vi "Online Spectrogram Monitoring (DAQmx).vi"() -> ()   [LabVIEW 2023]
doc: "This example shows how to configure a DAQ device, continuously acquire data from the specified physical channel with given sampling rate, and compute the real-time STFT spectrogram with the TFA Online STFT Spectrogram VI.\n\n<b>Requirements:</b>\nThis example requires a DAQ device and NI-DAQmx driver.\n\n<b>Instructions:</b>\n1) Select the data acquisition channel and sampling rate.\n2) Set the parameters for the STFT.\n3) Run this VI.\n4) Observe what frequencies are in your signal from the spectrogram.\n5) Browse the Block Diagram to learn how to configure the charts and how to connect TFA VIs with DAQmx VIs."
uses:
  <vilib>/DAQmx/read.llb/DAQmx Read (Analog 1D DBL 1Chan NSamp).vi
  <vilib>/DAQmx/create/channels.llb/DAQmx Create Channel (AI-Acceleration-Accelerometer).vi
  <vilib>/DAQmx/configure/timing.llb/DAQmx Timing (Sample Clock).vi
  <vilib>/DAQmx/miscellaneous.llb/DAQmx Fill In Error Info.vi
  <vilib>/addons/Time Frequency Analysis/Spectrogram.llb/TFA Online STFT Spectrogram (Real).vi
  <vilib>/addons/Time Frequency Analysis/_control.llb/TFA Configure Spectrogram Indicator (Predefined Color Table).vi
  <vilib>/addons/_Advanced Signal Processing/NI_AdvSigProcTFA.lvlib
  <resource>/objmgr/daqmx.rc
panel:
  out "aspt-left-top":bool
  in  "Window info":cluster{"type":u16, "length":i32}={"type"=0, "length"=256} {"type" items=["None ", "Hanning", "Hamming", "Blackman-Harris", "Exact Blackman", "Blackman", "Flat Top", "4 Term B-Harris ", "7 Term B-Harris", "Low Sidelobe", "Gaussian"]}
  in  "dB?":bool
  in  "Stop":bool
  in  "Sampling rate (Hz)":dbl=10000.0 format="%.2f"
  in  "Channel":tag="Dev2/ai0"
  in  "Frequency bins":i32=512
  in  "Time steps":i32=64
  out "Signal":dbl[](graph)
  out "Spectrogram":dbl[][](graph)
  # "Overview: Shows how to configure a DAQ device,  continuously acquire data from the specified physical channel with given sampling rate, and compute the real-time STFT spectrogram with the TFA Online STFT Spectrogram VI.\nRequirements: LabVIEW Full Development System, Advanced Signal Processing Toolkit, DAQmx Device\nInstructions: \n1. Select the data acquisition channel and sampling rate.\n2. Set the parameters for the STFT.\n3. Run this VI.\n4. Observe what frequencies are in your signal from the spectrogram.\n5. Browse the block diagram to learn how to configure the charts and how to connect TFA VIs with DAQmx VIs.\n6. Click Stop to stop the VI."
  # "Hardware Settings"
  # "Signal and Spectrogram"
  # "STFT Settings"
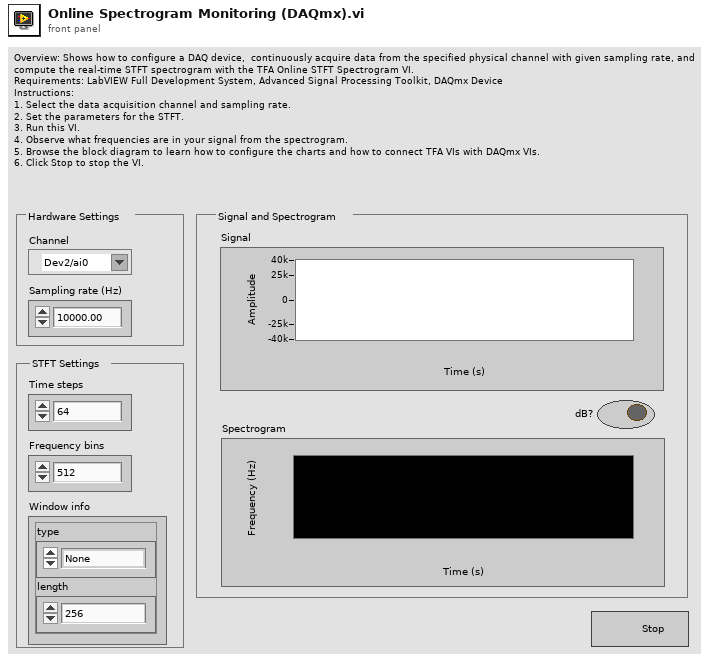
[diagram p1: front panel]
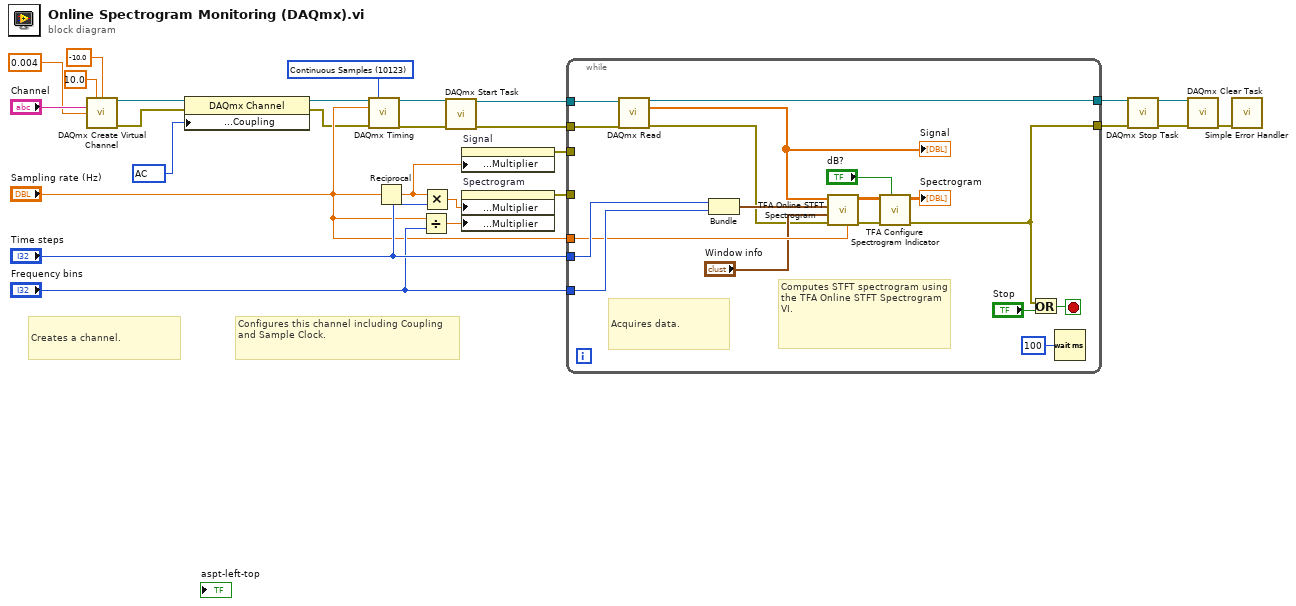
[diagram p0: block diagram]
diagram:
  w1 = 10045 items=["AC"=10045, "DC"=10050, "GND"=10066] ("AI.Coupling")
  w24 = 10123 items=["Finite Samples"=10178, "Continuous Samples"=10123, "Hardware Timed Single Point"=12522] ("sample mode")
  # "Configures this channel including Coupling and Sample Clock."
  # "Creates a channel."
  n1 = call-poly <vilib>:"DAQmx Create Virtual Channel.vi"("maximum value"=10.0, "minimum value"=-10.0, "physical channels"="Channel", "current excitation value"=0.004) -> ("task out"=w8:refnum<k21>, "error out"=w6:errorcluster)  [unwired: 9 in, 1 out]
  n2 = property class="DAQmx Channel"(reference=w8, error in=w6, "Analog Input:General Properties:Input Configuration:Coupling"=w1) -> (reference out=w7:refnum<k21>, error out=w5:errorcluster)
  n3 = call-poly <vilib>:"DAQmx Timing.vi"("task/channels in"=w7, "sample mode"=w24, "rate"="Sampling rate (Hz)", "error in"=w5) -> ("task out"=w26:refnum<k21>, "error out"=w25:errorcluster)  [unwired: 3 in, 7 out]
  n4 = Reciprocal(x="Sampling rate (Hz)") -> (1/x=w16:dbl)
  n5 = Divide(x="Sampling rate (Hz)", y="Frequency bins") -> (x/y=w18:dbl)
  n6 = Multiply(x=w16, y="Time steps") -> (x*y=w17:dbl)
  n7 = call <vilib>:"DAQmx Start Task.vi"("task/channels in"=w26, "error in"=w25) -> ("task out"=w23:refnum<k21>, "error out"=w22:errorcluster)  [unwired: 12 out]
  n8 = property on="Signal" class="WFChart (strict)"("X Scale.Offset and Multiplier:Multiplier"=w16) -> (error out=w15:errorcluster)  [unwired: 2 in, 1 out]
  n9 = property on="Spectrogram" class="IntChart (strict)"("X Scale.Offset and Multiplier:Multiplier"=w17, "Y Scale.Offset and Multiplier:Multiplier"=w18) -> (error out=w14:errorcluster)  [unwired: 2 in, 1 out]
  n10 = while {
    tunnel: w23 -> [w45]
    tunnel: w22 -> [w44]
    tunnel: [w42] -> w21
    tunnel: w15 -> [_]
    tunnel: w14 -> [_]
    tunnel: "Time steps" -> [w37]
    tunnel: "Frequency bins" -> [w36]
    tunnel: "Sampling rate (Hz)" -> [w35]
    tunnel: [w29] -> w2
    stop <- w32 stop-if-true
    # "Computes STFT spectrogram using the TFA Online STFT Spectrogram VI."
    # "Acquires data."
    n11 = call-poly <vilib>:"DAQmx Read.vi"("task/channels in"=w45, "error in"=w44) -> ("task out"=w42:refnum<k21>, "data"=w41:dbl[], "error out"=w30:errorcluster)  [unwired: 1 in, 10 out]
    "Signal" <- w41
    n12 = Bundle("Time steps"=w37, "Frequency bins"=w36) -> (w40:cluster{"Time steps":i32, "Frequency bins":i32})  [unwired: 1 out]
    n13 = call-poly <vilib>:"TFA Online STFT Spectrogram.vi"("sampling rate"=w35, "error in (no error)"=w30, "window info"="Window info", "time-frequency sampling info"=w40, "signal"=w41) -> ("error out"=w31:errorcluster, "spectrogram"=w39:dbl[][])  [unwired: 1 in, 4 out]
    n14 = call-poly <vilib>:"TFA Configure Spectrogram Indicator.vi"("dB on? (F)"="dB?", "error in (no error)"=w31, "spectrogram"=w39) -> ("error out"=w29:errorcluster, "TF spectrogram indicator"=→"Spectrogram":dbl[][])  [unwired: 4 in, 3 out]
    n15 = Or(x=w29, y="Stop") -> (x .or. y?=w32:bool)
    n16 = Wait (ms)(milliseconds to wait=u32 100) -> ()  [unwired: 1 out]
  }
  n17 = call <vilib>:"DAQmx Stop Task.vi"("task/channels in"=w21, "error in"=w2) -> ("task out"=w20:refnum<k21>, "error out"=w19:errorcluster)  [unwired: 12 out]
  n18 = call <vilib>:"DAQmx Clear Task.vi"("task in"=w20, "error in"=w19) -> ("error out"=w3:errorcluster)  [unwired: 13 out]
  n19 = call <vilib>:"Simple Error Handler.vi"("error in (no error)"=w3) -> ()  [unwired: 4 in, 5 out]
